vi "LIA_FPGA3a1.vi"() -> (1 "K Constant":fxp<+/-,32,16>, 2 "Nominal Freq":fxp<+/-,64,32>)   [LabVIEW 2012]
uses:
  <vilib>/Platform/TimedLoop/XDataNode/timing_clust.ctl
  <vilib>/Platform/TimedLoop/XDataNode/nitl_modes.ctl
  <vilib>/Platform/TimedLoop/XDataNode/wakeup.ctl
  <vilib>/rvi/DataTransferAndStorage/Container/Common/niFpgaContainerMetaDataKey.ctl
  <vilib>/rvi/DataTransferAndStorage/Container/Common/niFpgaContainerState.ctl
  <vilib>/rvi/DataTransferAndStorage/Container/Common/niFpgaDataTypeControl.ctl
  <vilib>/rvi/DataTransferAndStorage/Container/Common/niFpgaContainerImplementationControl.ctl
  <vilib>/rvi/DataTransferAndStorage/Container/Common/niFpgaContainerArbitrationOptionsControl.ctl
  <vilib>/rvi/DataTransferAndStorage/Container/Common/niFpgaTransferTypeControl.ctl
  <vilib>/rvi/DataTransferAndStorage/Container/Common/niFpgaContainerInitializationParameters.ctl
  <vilib>/rvi/Memory/Memory_Types/niFpgaMemoryInterfaceConfiguration.ctl
  <vilib>/rvi/FIFO/Fifo_Types/niFpgaFifoControlLogicControl.ctl
  <vilib>/rvi/eio/common/nirviEmuTemplateMethod_errors.vi
  <vilib>/rvi/Emulation/niFpgaSctlEmulationGetInTimedLoop.vi
  <vilib>/rvi/DataTransferAndStorage/Container/Common/niFpgaContainerGetUniqueNameForEmu.vi
  <vilib>/rvi/FIFO/Fifo_Resource/nirvififoEmulationSetSize.vi
  <vilib>/rvi/errors/niFpgaSetErrorForExecOnDevCompSimple.vi
  <vilib>/rvi/eio/common/nirviEmuReportErrorAndStop.vi
  <vilib>/rvi/Emulation/niFpgaSctlEmulationFifoFullMgr.vi
  <vilib>/rvi/Emulation/niFpgaSctlEmulationResourceMgr.vi
  <vilib>/rvi/Emulation/niFpgaSctlEmulationRegisterWithScheduler.vi
  <vilib>/rvi/Emulation/niFpgaSctlEmulationScheduler.vi
  <vilib>/rvi/DataTransferAndStorage/Container/Common/niFpgaContainerSetEmuInfo.vi
  <vilib>/eio/EIONode/EIONode.xnode
  <vilib>/Platform/TimedLoop/XDataNode/XDataNode.xnode
  <vilib>/rvi/FXPMathLib/FxpInterpret/XNode/nifxpmath_Interpret.xnode
  <vilib>/rvi/DataTransferAndStorage/Container/XNode/niFpgaContainer.xnode
  <vilib>/rvi/FIFO/Fifo_Resource/nirvififoEmulationWrite.vi
  <vilib>/rvi/FIFO/Fifo_Resource/nirvififoEmulationRead.vi
  <vilib>/rvi/LocalResourceManager/LocalResourceManager.xnode
  <vilib>/Platform/TimedLoop/XDataNode/XDNodeRunTimeDep.lvlib
panel:
  in  "Reference Signal":u64
  in  "VCO Sinz Output":u64
  in  "Period":u16=1000
  out "ticks":u16
  out "ref":i16 format="%.0x"
  out "sig":i16 format="%.0x"
  out "channelQ":i64
  out "channelI":i64
  out "f":fxp<+/-,32,0> format="%.32g"
  in  "dec2":i16=1
  in  "K":fxp<+,16,0>=0.001007080078125
  in  "nominal freq":fxp<+,16,0>=0.010009765625
  in  "dec1":i16=1
  in  "stages":i8=1
  in  "stop":bool
  in  "decimation":i16=1024
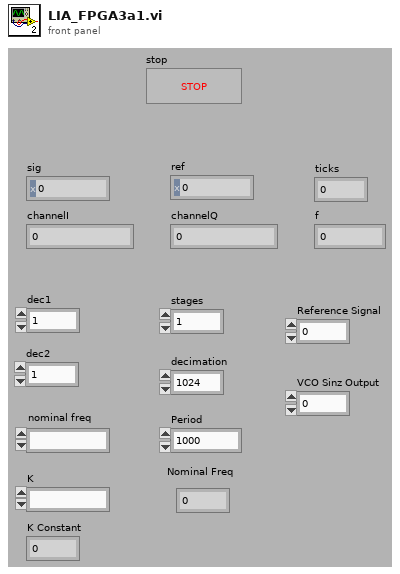
[diagram p1: front panel]
types:
  T1 = typedef "XDNodeRunTimeDep.lvlib/timing_clust.ctl" = cluster{"Expected End [f-1]":u64, "Actual End [f-1]":u64, "Finished Late? [f-1]":bool, "Expected End [i-1]":u64, "Actual End [i-1]":u64, "Finished Late? [i-1]":bool, "Expected Start [i]":u64, "Actual Start [i]":u64, "Expected Start [f]":u64, "Actual Start [f]":u64, "Source Name":string, "Structure Name":string, "Period":i64, "Deadline":i64, "Offset":i64, "Start":i64, "Priority":i32, "Timeout":i32, "Mode":T2, "Wakeup Reason":T3, "Error":errorcluster, "Source Type":string, "Secondary Source Type":string, "Global End Time":u64, "Global Start Time":u64, "Frame Duration":u64, "Iteration Duration":u64, "Assigned CPU":i32, "I/O Scan Engine Mode":u32}
  T2 = typedef "XDNodeRunTimeDep.lvlib/nitl_modes.ctl" = enum32{"No Change", "Process missed periods, maintain original phase", "Discard missed periods, maintain original phase", "Process missed periods, ignore original phase", "Discard missed periods, ignore original phase"}
  T3 = typedef "XDNodeRunTimeDep.lvlib/wakeup.ctl" = enum32{"Normal", "Aborted", "Asynchronous wakeup", "Timing source error", "Timed loop error", "Timeout"}
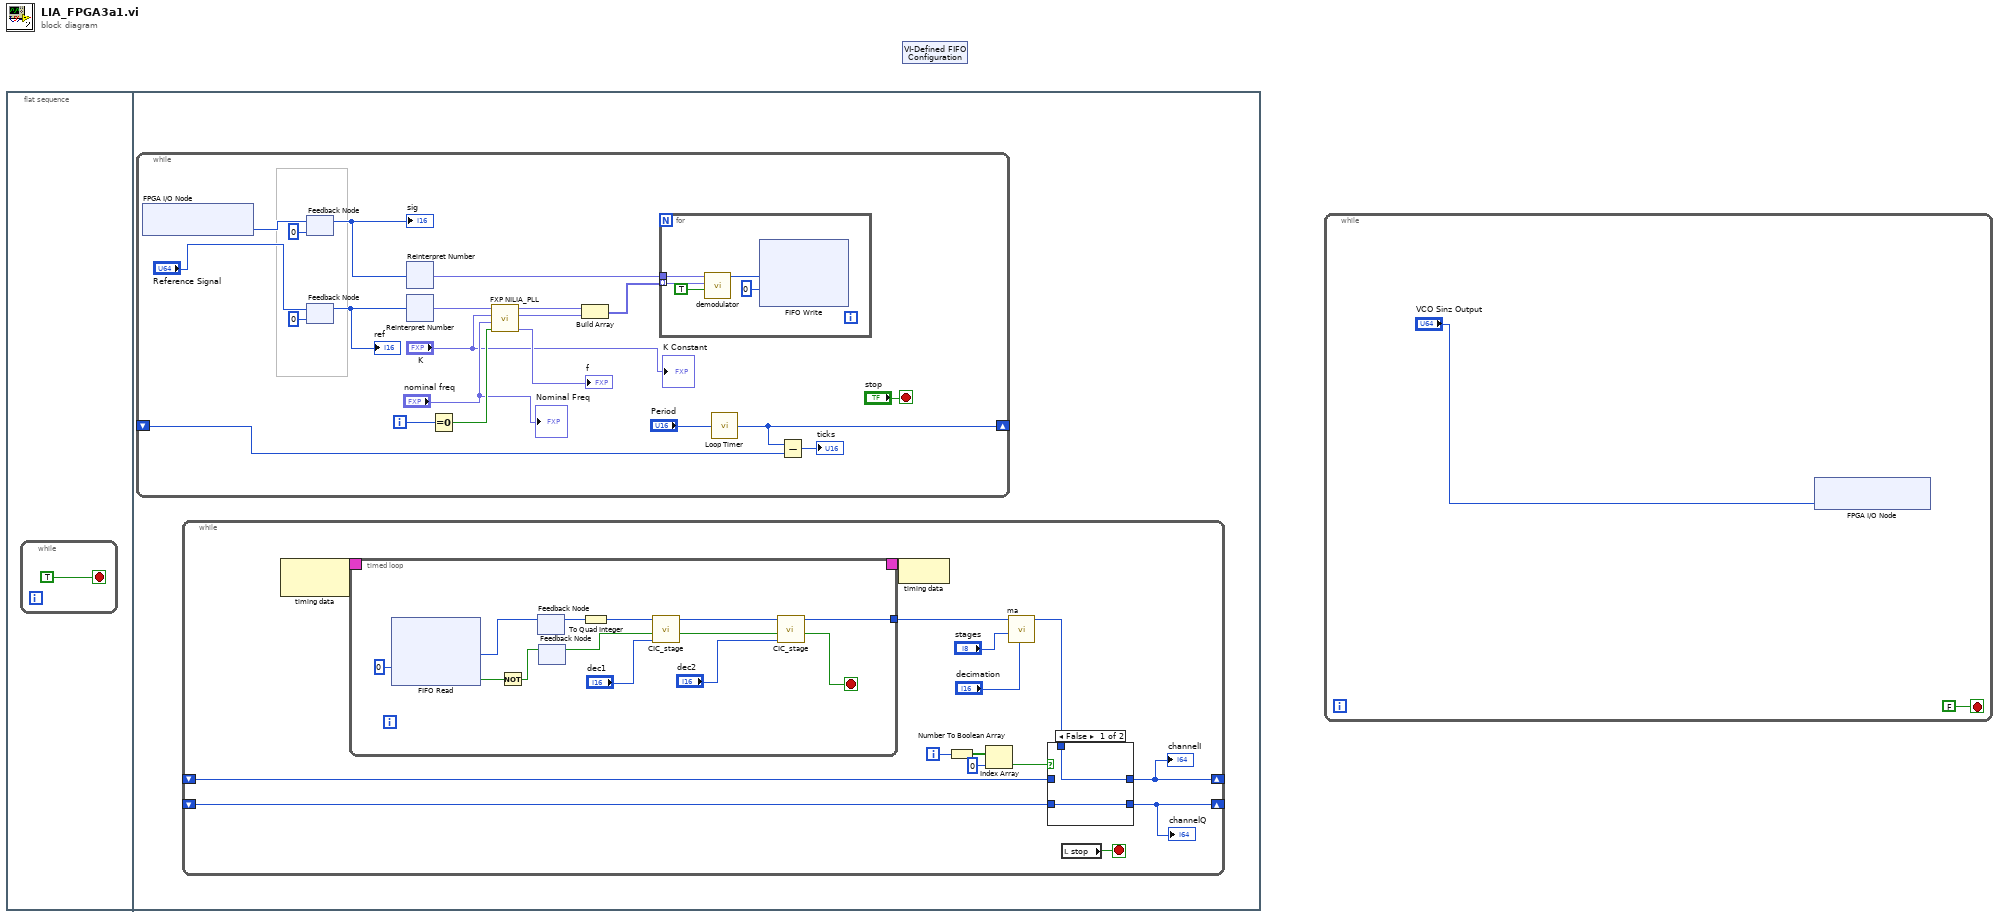
[diagram p0: block diagram]
diagram:
  n1 = flat-sequence {
    frame #0 {
      n2 = while {
        stop <- TRUE ("start") stop-if-true
      }
    }
    frame #1 {
      n3 = while {
        shift-right: [w19] -> _
        shift-left: _ -> [w18]
        i -> [w22]
        stop <- "stop" stop-if-true
        n4 = xnode "FPGA I/O Node"() -> ("Connector0/AI6"=w12:i16)  [unwired: 1 in, 1 out]
        n5 = feedback #1(i16 0 ("y")) -> (w11:i16)
        "sig" <- w11
        n6 = feedback-in #1(w12) -> ()
        n7 = feedback #2(i16 0 ("z [I32.1]")) -> (w10:u64)
        "ref" <- w10
        n8 = feedback-in #2("Reference Signal") -> ()
        n9 = xnode "Reinterpret Number"("x"=w11) -> ("y"=w15:fxp<+/-,16,1>)
        n10 = xnode "Reinterpret Number"("x"=w10) -> ("y"=w9:fxp<+/-,64,1>)
        n11 = Equal To 0?(x=w22) -> (x = 0?=w5:bool)
        n12 = call "FXP NILIA_PLL.vi"("reset?"=w5, "norminal freq [U16.0]"="nominal freq", "alpha [U16.0]"="K", "x[I16.1]"=w9) -> ("f"=→"f":fxp<+/-,32,0>, "sin(z)"=w7:fxp<+/-,16,2>, "cos(z)"=w6:fxp<+/-,16,2>)  [unwired: 4 in, 1 out]
        n13 = Build Array(w6, w7) -> (w16:fxp<+/-,16,2>[])
        n14 = for {
          tunnel: w15 -> [w25]
          tunnel: w16 -> [w23] mode=indexing
          n15 = call "demodulator.vi"("New Data"=TRUE, "ref"=w23, "signal"=w25) -> ("x*y"=w26:i32)  [unwired: 8 out]
          n16 = xnode ("FIFO Write")("Element"=w26, "Timeout"=0) -> ()  [unwired: 1 in, 2 out]
        }
        n17 = call "Loop Timer"("Count(Ticks)"="Period") -> ("Tick Count(Ticks)"=w19:u16)
        n18 = Subtract(x=w19, y=w18) -> (x-y=→"ticks":u16)
        "Nominal Freq" <- "nominal freq"
        "K Constant" <- "K"
      }
      n19 = while {
        shift-right: [w29] -> _
        shift-left: _ -> [w31]
        shift-right: [w28] -> _
        shift-left: _ -> [w30]
        i -> [w36]
        stop <- w38 stop-if-true
        n20 = node-c288() -> (w42:T1)  [unwired: 1 out]
        n21 = timed-loop {
          timing: w42 -> [_]
          timing-out: [_] -> w41
          tunnel: [w50] -> w37
          stop <- w49 stop-if-true
          n22 = xnode ("FIFO Read")("Timeout"=0) -> ("Element"=w57:i32, "Timed Out?"=w56:bool)  [unwired: 1 in, 1 out]
          n23 = Not(x=w56) -> (.not. x?=w55:bool)
          n24 = feedback-in #3(w57) -> ()
          n25 = feedback #3() -> (w59:i32)  [unwired: 1 out]
          n26 = feedback-in #4(w55) -> ()
          n27 = feedback #4() -> (w53:bool)  [unwired: 1 out]
          n28 = To Quad Integer(1:w59) -> (0:w54:i64)
          n29 = call "CIC_stage.vi"("decimate factor"="dec1", "New Data"=w53, "input"=w54) -> ("Data Ready"=w51:bool, "output"=w52:i64)  [unwired: 7 out]
          n30 = call "CIC_stage.vi"("decimate factor"="dec2", "New Data"=w51, "input"=w52) -> ("Data Ready"=w49:bool, "output"=w50:i64)  [unwired: 7 out]
        }
        n31 = node-c288(w41) -> ()
        n32 = Number To Boolean Array(number=w36) -> (Boolean array=w35:bool[])
        n33 = Index Array "Index Array"(array=w35, index=0) -> (element=w33:bool)
        n34 = call "ma.vi"("decimate"="decimation", "stages"="stages", "input"=w37) -> ("output"=w32:i64)  [unwired: 8 out]
        n35 = case shown="False" w33 {
          tunnel: w32 -> [w44 w46]
          tunnel: [w44 w45] -> w29
          tunnel: [w43 w46] -> w28
          tunnel: w31 -> [_ w45]
          tunnel: w30 -> [w43 _]
          frame False {
          }
          frame True {
          }
        }
        "channelI" <- w29
        "channelQ" <- w28
        n36 = local read "stop"() -> (w38:bool)
      }
    }
  }
  n37 = xnode "VI-Defined FIFO Configuration"() -> ()  [unwired: 1 out]
  n38 = while {
    stop <- FALSE stop-if-true
    n39 = xnode "FPGA I/O Node"("Connector0/AO5"="VCO Sinz Output") -> ()  [unwired: 1 in, 1 out]
  }
